vi "2D DBL to 2D String.vi"(8 "error in (no error)":errorcluster, 11 "Data":dbl[][](array[numeric])) -> (0 "error out":errorcluster, 1 "# of Columns":i32, 2 "# of Rows":i32, 3 "Table":string[][](table))   [LabVIEW 2019, in "Table Tools.lvlib"]
doc: "Convert 2D-Double to 2-D String for tables."
uses:
  Table Tools.lvlib
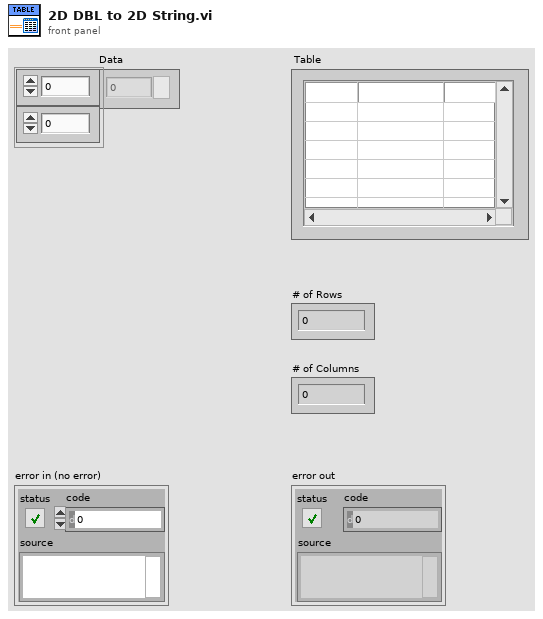
[diagram p1: front panel]
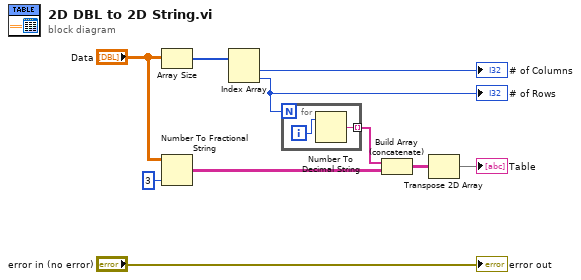
[diagram p0: block diagram]
diagram:
  n1 = Array Size(array="Data") -> (size(s)=w9:i32[])
  n2 = Number To Fractional String(number="Data", precision (6)=i16 3) -> (F-format string=w8:string[][])  [unwired: 2 in]
  n3 = Index Array(array=w9) -> (element #1=→"# of Columns":i32, element #2=w5:i32)  [unwired: 2 in]
  "# of Rows" <- w5
  n4 = for {
    N: w5 -> [_]
    tunnel: [w11] -> w4 mode=indexing
    i -> [w12]
    n5 = Number To Decimal String(number=w12) -> (decimal integer string=w11:string)  [unwired: 1 in]
  }
  n6 = Build Array (concatenate)(w4, w8) -> (w6:string[][])
  n7 = Transpose 2D Array(2D array=w6) -> (transposed array=→"Table":string[][])
  "error out" <- "error in (no error)"
